vi "Draw Lines.vi"(4 "wheel frame angle (rad)":dbl, 6 "color (black)":u32(colorbox), 7 "picture info":T1={"picture size"={"Width"=500, "Height"=500}, "pixels per unit"=10.0}, 8 "end points":cluster{"x":dbl, "y":dbl}[](array[cluster]), 9 "start points":cluster{"x":dbl, "y":dbl}[](array[cluster]), 10 "global wheel position":cluster{"x":dbl, "y":dbl}, 11 "picture in":picture) -> (3 "picture out":picture)   [LabVIEW 2017, in "NI_Robotics_Steering Picture.lvlib"]
uses:
  <vilib>/robotics/Utilities/Visualization/Steering Visualization/Steering Picture/NI_Robotics_Steering Picture.lvlib
  <vilib>/robotics/Utilities/Visualization/Steering Visualization/Steering Picture/Picture Info.ctl
  <vilib>/Utility/miscctls.llb/LVBoundsTypeDef.ctl
  <vilib>/Analysis/coordinate.llb/2D Cartesian Coordinate Rotation (Array).vi
  <vilib>/Analysis/NI_AALPro.lvlib
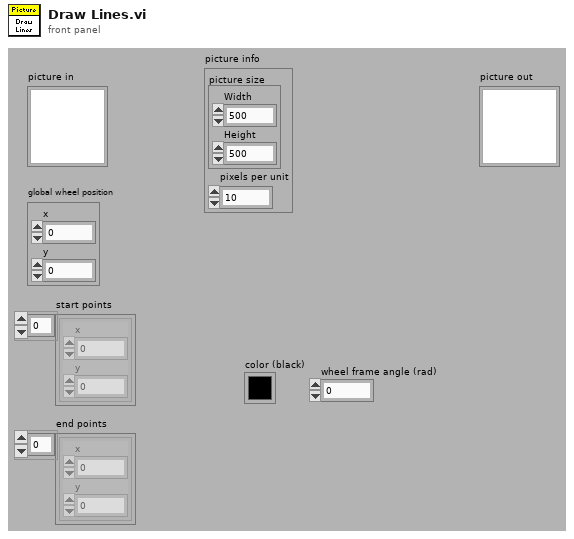
[diagram p1: front panel]
types:
  T1 = typedef "NI_Robotics_Steering Picture.lvlib/Picture Info.ctl" = cluster{"picture size":T2, "pixels per unit":dbl}
  T2 = typedef "LVBoundsTypeDef.ctl" = cluster{"Width":u32, "Height":u32}
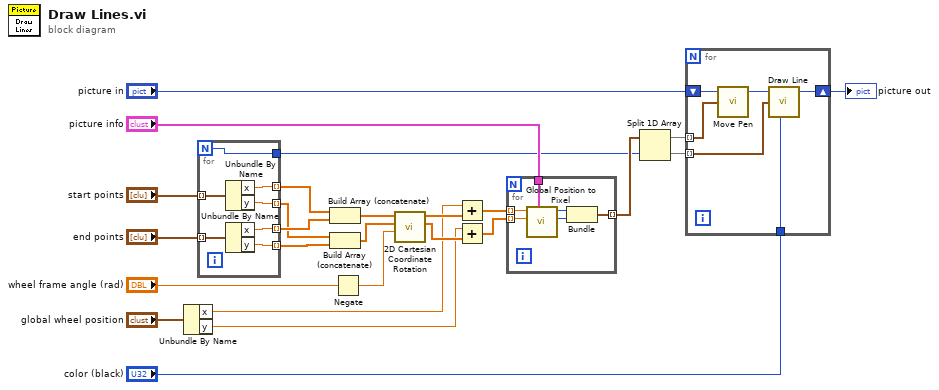
[diagram p0: block diagram]
diagram:
  n1 = Unbundle By Name("global wheel position") -> ("x"=w20:dbl, "y"=w19:dbl)
  n2 = for {
    N -> [w26]
    tunnel: "end points" -> [w31] mode=indexing
    tunnel: "start points" -> [w32] mode=indexing
    tunnel: [w30] -> w16 mode=indexing
    tunnel: [w29] -> w14 mode=indexing
    tunnel: [w28] -> w15 mode=indexing
    tunnel: [w27] -> w13 mode=indexing
    tunnel: [w26] -> w6
    n3 = Unbundle By Name(w32) -> ("x"=w30:dbl, "y"=w29:dbl)
    n4 = Unbundle By Name(w31) -> ("x"=w28:dbl, "y"=w27:dbl)
  }
  n5 = Build Array (concatenate)(w16, w15) -> (w12:dbl[])
  n6 = Build Array (concatenate)(w14, w13) -> (w11:dbl[])
  n7 = Negate(x="wheel frame angle (rad)") -> (-x=w9:dbl)
  n8 = call-poly <vilib>:"2D Cartesian Coordinate Rotation.vi"("theta"=w9, "Y"=w11, "X"=w12) -> ("Y Out"=w23:dbl[], "X Out"=w21:dbl[])  [unwired: 6 in, 1 out]
  n9 = Add(x=w20, y=w21) -> (x+y=w22:dbl[])
  n10 = Add(x=w19, y=w23) -> (x+y=w24:dbl[])
  n11 = for {
    tunnel: w22 -> [w38] mode=indexing
    tunnel: w24 -> [w37] mode=indexing
    tunnel: [w34] -> w7 mode=indexing
    tunnel: "picture info" -> [w33]
    n12 = call <vilib>:"Global Position to Pixel.vi"("picture info"=w33, "global y"=w37, "global x"=w38) -> ("pixel y"=w35:i16, "pixel x"=w36:i16)  [unwired: 7 in]
    n13 = Bundle("pixel x"=w36, "pixel y"=w35) -> (w34:cluster{"pixel x":i16, "pixel y":i16})  [unwired: 1 in]
  }
  n14 = Split 1D Array(array=w7, index=w6) -> (first subarray=w5:cluster{"pixel x":i16, "pixel y":i16}[], second subarray=w4:cluster{"pixel x":i16, "pixel y":i16}[])
  n15 = for {
    tunnel: w5 -> [w43] mode=indexing
    tunnel: w4 -> [w41] mode=indexing
    shift-right: [w40] -> w2
    shift-left: "picture in" -> [w44]
    tunnel: "color (black)" -> [w39]
    n16 = call <vilib>:"Move Pen.vi"("new position"=w43, "picture"=w44) -> ("new picture"=w42:picture)  [unwired: 3 in]
    n17 = call <vilib>:"Draw Line.vi"("picture"=w42, "end point"=w41, "color(black)"=w39) -> ("new picture"=w40:picture)  [unwired: 6 in]
  }
  "picture out" <- w2
